vi "deflection control.vi"() -> ()   [LabVIEW 2017]
uses:
  <vilib>/rvi/Emulation/niFpgaGetClockAttributes.vi
  <vilib>/rvi/Emulation/niFpgaSctlEmulationGetInTimedLoop.vi
  <vilib>/rvi/Emulation/niFpgaEmulationReportErrorSimple.vi
  <vilib>/rvi/eio/common/nirviEmuTemplateMethod_errors.vi
  <vilib>/rvi/Emulation/niFpgaCriticalErrorInLSC.vi
  <vilib>/eio/EIONode/EIONode.xnode
  <vilib>/rvi/FXPMathLib/FxpSub/XNode/nifxpmath_Sub.xnode
  <vilib>/rvi/FXPMathLib/FxpMul/XNode/nifxpmath_Multiplier.xnode
  <vilib>/rvi/FXPMathLib/FxpAdd/XNode/nifxpmath_Add.xnode
  <vilib>/rvi/FXPMathLib/sim/FxpSim.dll
panel:
  in  "Lower Limit":fxp<+/-,64,29>
  in  "Upper Limit":fxp<+/-,64,29>
  in  "P":fxp<+/-,20,5>
  in  "I":fxp<+/-,20,5>
  in  "SetPoint":fxp<+/-,20,5>
  in  "stop":bool
  out "Mod1/AI2":fxp<+/-,20,5>
  out "Output":fxp<+/-,64,29>
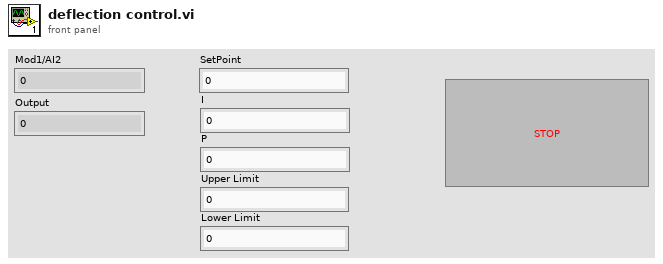
[diagram p1: front panel]
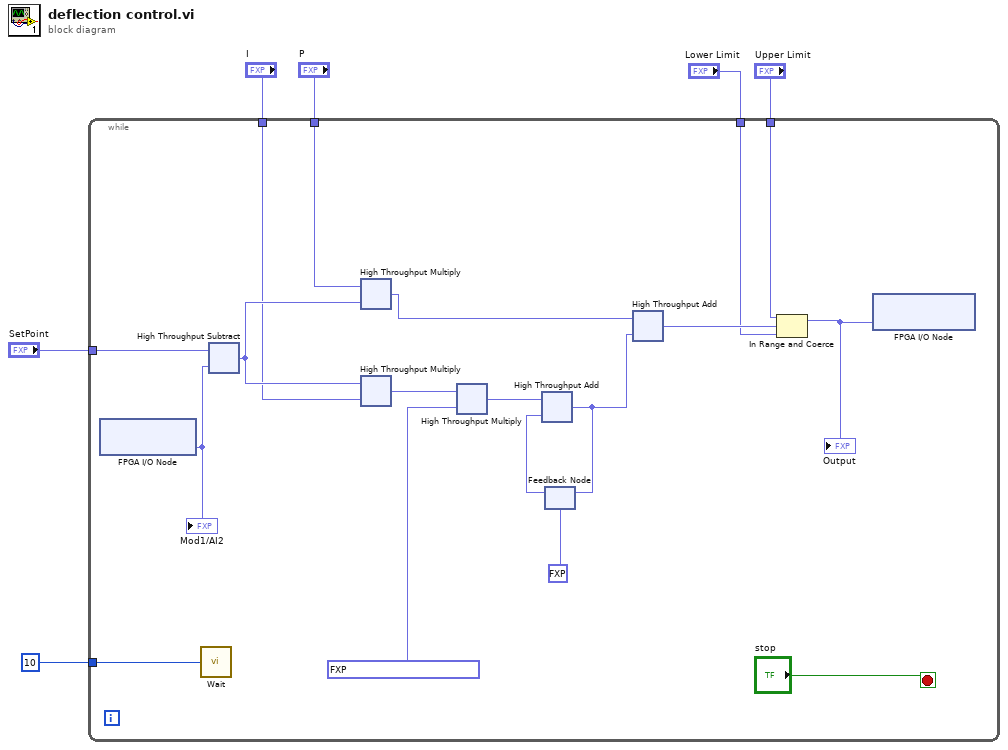
[diagram p0: block diagram]
diagram:
  n1 = while {
    tunnel: "SetPoint" -> [w23]
    tunnel: "P" -> [w22]
    tunnel: "I" -> [w20]
    tunnel: u32 10 ("Count(uSec)") -> [w18]
    tunnel: "Upper Limit" -> [w10]
    tunnel: "Lower Limit" -> [w9]
    stop <- "stop" stop-if-true
    n2 = xnode "FPGA I/O Node"() -> ("Mod1/AI3"=w7:fxp<+/-,20,5>)  [unwired: 1 in, 1 out]
    "Mod1/AI2" <- w7
    n3 = call "Wait"("Count(uSec)"=w18) -> ()  [unwired: 1 out]
    n4 = xnode ("High Throughput Subtract")("x"=w23, "y"=w7) -> ("x-y"=w21:fxp<+/-,21,6>)
    n5 = xnode ("High Throughput Multiply")("x"=w22, "y"=w21) -> ("x*y"=w13:fxp<+/-,41,11>)
    n6 = xnode ("High Throughput Multiply")("x"=w21, "y"=w20) -> ("x*y"=w19:fxp<+/-,41,11>)
    n7 = xnode ("High Throughput Multiply")("x"=w19, "y"=fxp<+/-,32,5> 9.998679161071777e-06) -> ("x*y"=w16:fxp<+/-,64,16>)
    n8 = feedback #1(fxp<+,1,1> 0.0) -> (w14:fxp<+/-,64,28>)
    n9 = xnode ("High Throughput Add")("x"=w16, "y"=w14) -> ("x+y"=w12:fxp<+/-,64,28>)
    n10 = feedback-in #1(w12) -> ()
    n11 = xnode ("High Throughput Add")("x"=w13, "y"=w12) -> ("x+y"=w11:fxp<+/-,64,29>)
    n12 = In Range and Coerce(upper limit=w10, x=w11, lower limit=w9) -> (coerced(x)=w8:fxp<+/-,64,29>)  [unwired: 1 out]
    "Output" <- w8
    n13 = xnode "FPGA I/O Node"("Mod8/AO2"=w8) -> ()  [unwired: 1 in, 1 out]
  }
